vi "MGCC_FntStaMach_PV_control.vi"   [LabVIEW 2016]
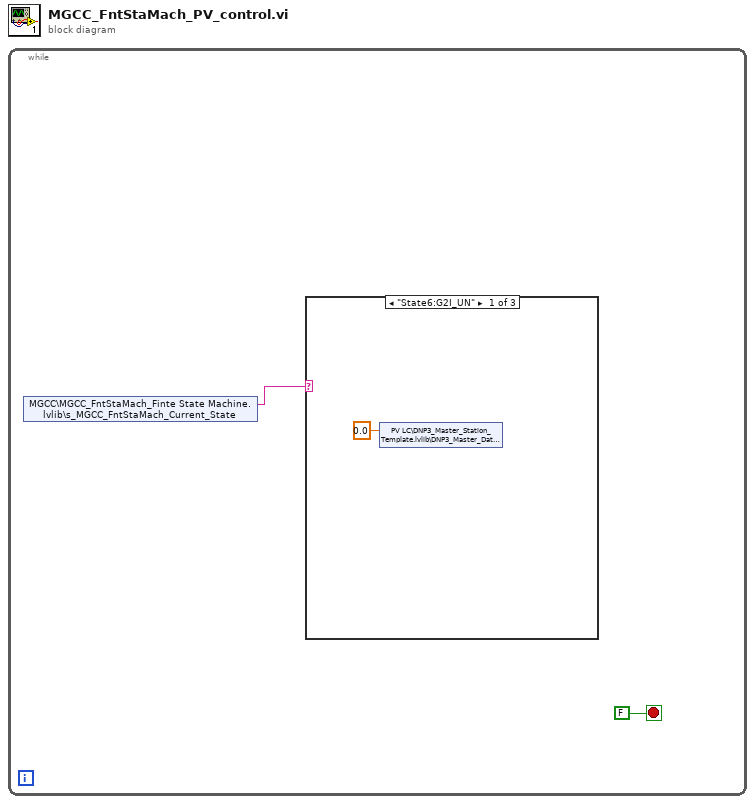
[diagram p0: block diagram]
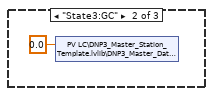
[diagram p2: hidden frame]
diagram:
  n1 = while {
    stop <- FALSE stop-if-true
    n2 = shared-variable "MGCC\\MGCC_FntStaMach_Finte State Machine.lvlib\\s_MGCC_FntStaMach_Current_State"() -> (w1:string)  [unwired: 1 in, 1 out]
    n3 = case shown="\"State6:G2I_UN\"" w1 {
      frame "State6:G2I_UN" {
        n4 = shared-variable "PV LC\\DNP3_Master_Station_Template.lvlib\\DNP3_Master_Data_Variables.lvlib\\MS_Analog_Control.lvlib\\PV-RESERVED5"(0.0 ("PV-RESERVED5")) -> ()  [unwired: 1 in, 1 out]
      }
      frame "State3:GC" {
        n5 = shared-variable "PV LC\\DNP3_Master_Station_Template.lvlib\\DNP3_Master_Data_Variables.lvlib\\MS_Analog_Control.lvlib\\PV-RESERVED5"(0.0 ("PV-RESERVED5")) -> ()  [unwired: 1 in, 1 out]
      }
      frame "State6:G2I_IN", Default {
      }
    }
  }
